vi "1-2.vi"() -> ()   [LabVIEW 2022 SP3, in "AoC22.lvlib"]
uses:
  AoC22.lvlib
  5aa7e717-9c48-40ee-8198-4254aee5384a.vi
  <vilib>/Comparison/Less/Less Functor/Less Functor.lvclass
panel:
  out "sum":i32
  out "string array":string[](array[string])
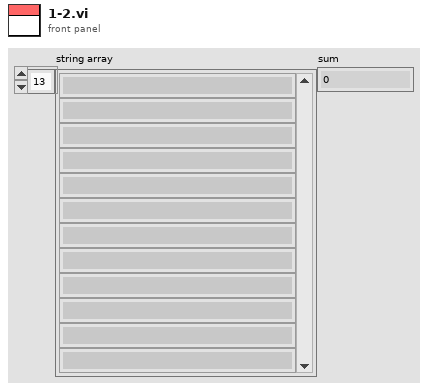
[diagram p1: front panel]
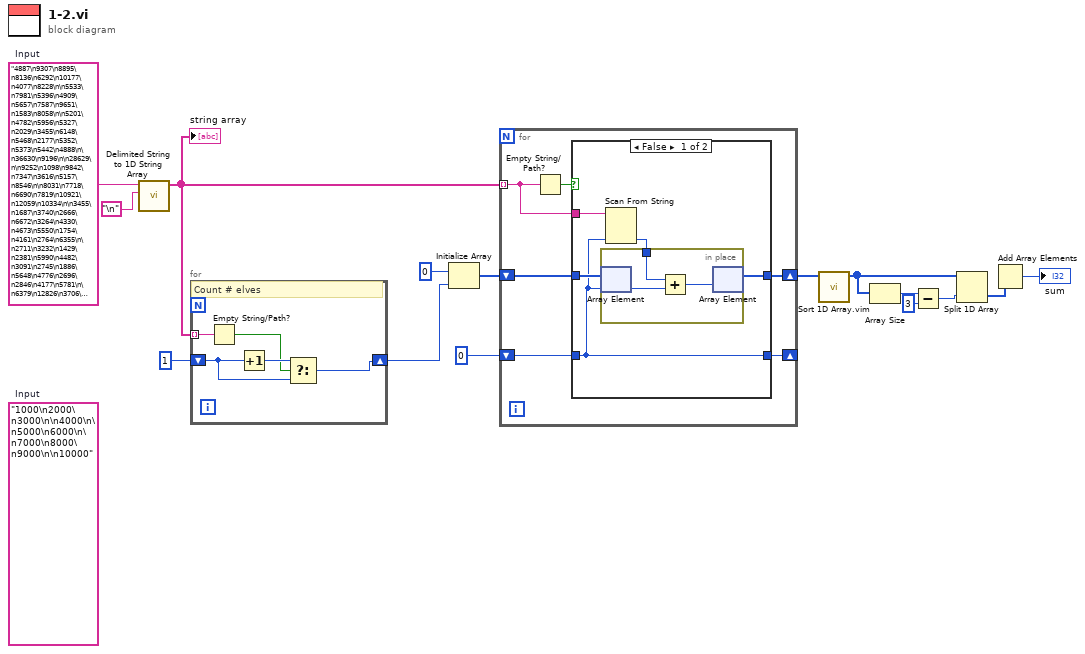
[diagram p0: block diagram]
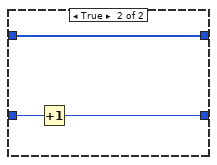
[diagram p2: hidden frame]
diagram:
  (unwired) "1000\n2000\n3000\n\n4000\n\n5000\n6000\n\n7000\n8000\n9000\n\n10000"  # Input
  w13 = "4887\n9307\n8895\n8136\n6292\n10177\n4077\n8228\n\n5533\n7981\n5396\n4909\n5657\n7587\n9651\n1583\n8058\n\n5201\n4782\n5956\n5327\n2029\n3455\n6148\n5468\n2177\n5352\n5373\n5442\n4888\n\n36630\n9196\n\n28629\n\n9252\n1098\n9842\n7347\n3616\n5157\n8546\n\n8031\n7718\n6690\n7819\n10921\n12059\n10334\n\n3455\n1687\n3740\n2666\n6672\n3264\n4330\n4673\n5550\n1754\n4161\n2764\n6355\n\n2711\n3232\n1429\n2381\n5990\n4482\n3091\n2745\n1886\n5648\n4776\n2696\n2846\n4177\n5781\n\n6379\n12826\n3706\n12650\n5875\n11396\n\n10381\n2204\n5950\n11465\n11501\n13306\n\n4006\n6635\n5139\n5290\n4562\n5558\n2788\n1242\n5308\n6704\n6858\n3751\n\n3574\n5601\n4492\n4795\n2135\n3295\n6150\n4786\n6761\n5098\n6646\n5839\n1989\n\n14468\n13500\n11..."  # Input
  n1 = call <vilib>:"Delimited String to 1D String Array.vi"("delimiter"="\n", "delimited string"=w13) -> ("string array"=w10:string[])  [unwired: 9 in]
  "string array" <- w10
  n2 = for {
    tunnel: w10 -> [w20] mode=indexing
    shift-right: [w19] -> w12
    shift-left: 1 -> [w18]
    # "Count # elves"
    n3 = Empty String/Path?(string/path=w20) -> (empty?=w16:bool)
    n4 = Increment(x=w18) -> (x+1=w17:i32)
    n5 = Select(t=w17, s=w16, f=w18) -> (s? t:f=w19:i32)
  }
  n6 = Initialize Array(0 ("element"), w12) -> (w9:i32[])
  n7 = for {
    tunnel: w10 -> [w25] mode=indexing
    shift-right: [w21] -> w7
    shift-left: w9 -> [w23]
    shift-right: [w22] -> _
    shift-left: 0 -> [w24]
    n8 = Empty String/Path?(string/path=w25) -> (empty?=w26:bool)
    n9 = case shown="False" w26 {
      tunnel: w25 -> [w29 _]
      tunnel: w24 -> [w28 w37]
      tunnel: w23 -> [w31 w35]
      tunnel: [w28 w36] -> w22
      tunnel: [w30 w35] -> w21
      frame False {
        n10 = Scan From String(input string=w29, default 1=w28) -> (output 1=w27:i32)  [unwired: 3 in, 3 out]
        n11 = in-place {
          in-place-border: w27 -> [w32]
          n12 = in-place-array #1(w31, w28) -> (w34:i32)
          n13 = Add(x=w32, y=w34) -> (x+y=w33:i32)
          n14 = in-place-array #1(w33) -> (w30:i32[])  [unwired: 1 out]
        }
      }
      frame True {
        n15 = Increment(x=w37) -> (x+1=w36:i32)
      }
    }
  }
  n16 = call "Sort 1D Array.vim"("unsorted array"=w7) -> ("sorted array"=w4:i32[])  [unwired: 10 in]
  n17 = Array Size(array=w4) -> (size(s)=w3:i32)
  n18 = Subtract(x=w3, y=3) -> (x-y=w1:i32)
  n19 = Split 1D Array(array=w4, index=w1) -> (second subarray=w5:i32[])  [unwired: 1 out]
  n20 = Add Array Elements(numeric array=w5) -> (sum=→"sum":i32)
